vi "Do.vi"(8 "error in (no error)":errorcluster, 10 "Actor in":refnum<class "Actor.lvclass">, 11 "Configure Glitch Trigger Source [GT] Msg":refnum<class "Configure Glitch Trigger Source [GT] Msg.lvclass">) -> (0 "error out":errorcluster, 2 "Actor out":refnum<class "Actor.lvclass">)   [LabVIEW 2015, in "CS++Scope.lvlib" / "Configure Glitch Trigger Source [GT] Msg.lvclass"]
doc: "This VI delivers the message to the actor by calling the appropriate method(s) on the actor."
uses:
  Configure Glitch Trigger Source [GT] Msg.lvclass
  <vilib>/ActorFramework/Actor/Actor.lvclass
  CS++Scope/CS++Scope.lvclass
  Configure Glitch Trigger Source [GT] Msg.lvclass/Configure Glitch Trigger Source [GT] Msg.ctl
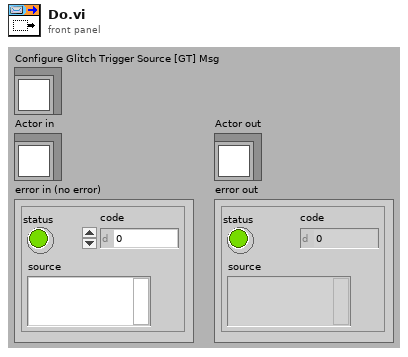
[diagram p1: front panel]
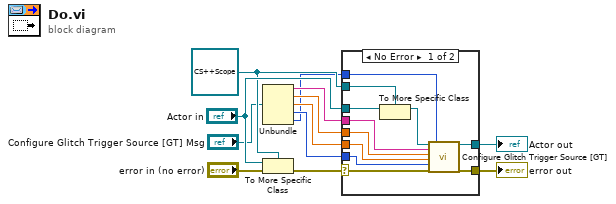
[diagram p0: block diagram]
diagram:
  w7 = refnum<class "CS++Scope.lvclass"> refnum ("Actor in")
  n1 = Unbundle ("Main-Unbundle")("Configure Glitch Trigger Source [GT] Msg") -> (w5:string, w4:dbl[unit], w3:dbl[unit], w2:i32, w1:i32)
  n2 = To More Specific Class(target class=w7, reference="Actor in", error in="error in (no error)") -> (error out=w11:errorcluster)  [unwired: 1 out]
  n3 = case shown="No Error" w11 {
    selector: w11 -> [w21 w25]
    tunnel: [w23 w25] -> w10
    tunnel: [w22 w24] -> w9
    tunnel: "Actor in" -> [w20 w24]
    tunnel: w7 -> [w19 _]
    tunnel: w5 -> [w17 _]
    tunnel: w4 -> [w16 _]
    tunnel: w3 -> [w15 _]
    tunnel: w2 -> [w14 _]
    tunnel: w1 -> [w13 _]
    frame No Error {
      n4 = To More Specific Class(target class=w19, reference=w20) -> (specific class reference=w18:refnum<class "CS++Scope.lvclass">)  [unwired: 1 in, 1 out]
      n5 = call "Configure Glitch Trigger Source [GT].vi"("CS++Scope"=w18, "trigger source (\"CHANNEL1\")"=w17, "trigger level (0.0 V)"=w16, "glitch width (10 ms)"=w15, "glitch polarity (Positive)"=w14, "error in (no error)"=w21, "glitch condition (Less Than)"=w13) -> ("CS++Scope out"=w22:refnum<class "CS++Scope.lvclass">, "error out"=w23:errorcluster)  [unwired: 11 in]
    }
    frame Error {
    }
  }
  "error out" <- w10
  "Actor out" <- w9
